vi "Open.vi"(4 "Gyro Full Scale Range":T8, 6 "Accel Full Scale Range":T9, 7 "I2C Channel":u8, 8 "error in (no error)":errorcluster, 9 "Clock Source":u8=1, 10 "Device Address":T10=104 items=["0x68"=104, "0x69"=105], 11 "LINX Resource":T1) -> (0 "error out":errorcluster, 3 "LINX Resource":T1)   [LabVIEW 2011, in "LINX-MPU60X0.lvlib"]
doc: "Initializes the MPU-60X0 device setting the clock source and the full ranges for the accelerometer and gyro."
uses:
  LINX-MPU60X0.lvlib
  AccelFullScaleRanges.ctl
  GyroFullScaleRanges.ctl
  <vilib>/LabVIEW Hacker/LINX/Private/Type Defs/Platform.ctl
  <vilib>/LabVIEW Hacker/LINX/Private/Type Defs/Interface.ctl
  <vilib>/LabVIEW Hacker/LINX/Private/Device/Type Defs/TCP Config.ctl
  <vilib>/LabVIEW Hacker/LINX/Private/Type Defs/Device Family.ctl
  <vilib>/LabVIEW Hacker/LINX/Private/Device/Type Defs/Channels.ctl
  <vilib>/LabVIEW Hacker/LINX/Private/Device/Type Defs/LINX Device Config.ctl
  <vilib>/LabVIEW Hacker/LINX/Private/Type Defs/LINX Ref.ctl
  DeviceAddresses.ctl
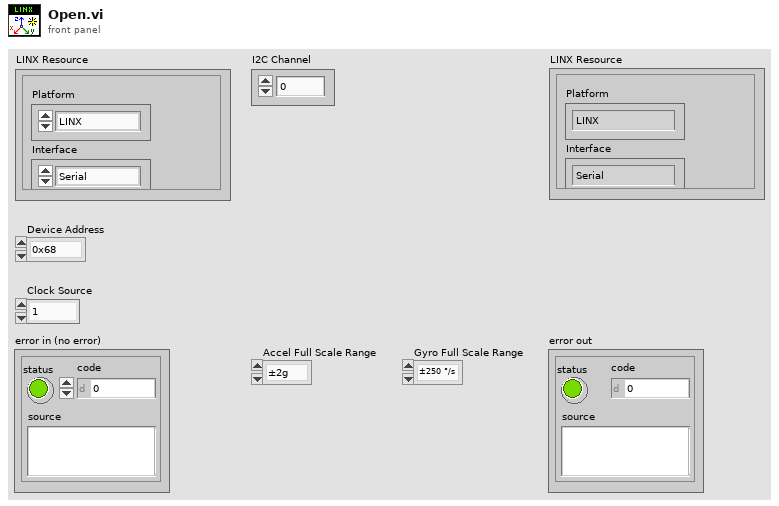
[diagram p1: front panel]
types:
  T1 = typedef "LVH-LINX.lvlib/LINX Ref.ctl" = cluster{"Platform":T2, "Interface":T3, "LINX Device Config":T4}
  T2 = typedef "LVH-LINX.lvlib/Platform.ctl" = enum16{"LINX", "myRIO"}
  T3 = typedef "LVH-LINX.lvlib/Interface.ctl" = enum16{"Serial", "TCP"}
  T4 = typedef "LVH-LINX.lvlib/Device.lvlib/LINX Device Config.ctl" = cluster{"Interface":T3, "COM Port":refnum<visa-resource-name>, "TCP Configuration":T5, "Device Family":T6, "Device ID":u8, "Device Name":string, "TCP Ref":refnum<k5>, "Channels":T7}
  T5 = typedef "LVH-LINX.lvlib/Device.lvlib/TCP Config.ctl" = cluster{"IP Address":string, "Port":u16}
  T6 = typedef "LVH-LINX.lvlib/Device Family.ctl" = enum8{"National Instruments", "Digilent", "Arduino"}
  T7 = typedef "LVH-LINX.lvlib/Channels.ctl" = cluster{"DI Channels":u8[], "DO Channels":u8[], "AI":u8[], "AO":u8[], "PWM":u8[], "QE":u8[], "UART":u8[], "I2C 2":u8[], "SPI":u8[], "CAN":u8[], "AI Ref (V)":dbl, "AO Resolution (Bits)":u8, "AO Ref (V)":dbl}
  T8 = typedef "LINX-MPU60X0.lvlib/GyroFullScaleRanges.ctl" = enum8{"±250 °/s", "±500 °/s", "±1000 °/s", "±2000 °/s"}
  T9 = typedef "LINX-MPU60X0.lvlib/AccelFullScaleRanges.ctl" = enum16{"±2g", "±4g", "±8g", "±16g"}
  T10 = typedef "LINX-MPU60X0.lvlib/DeviceAddresses.ctl" = u8
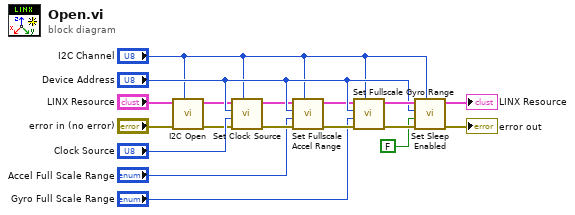
[diagram p0: block diagram]
diagram:
  n1 = call <vilib>:"I2C Open.vi"("I2C Channel (0)"="I2C Channel", "Error In"="error in (no error)", "LINX Resource"="LINX Resource") -> ("Error Out"=w2:errorcluster, "LINX Resource"=w4:T1)  [unwired: 7 in]
  n2 = call "Set Clock Source.vi"("I2C Channel"="I2C Channel", "error in (no error)"=w2, "Clock Source"="Clock Source", "Device Address"="Device Address", "LINX Resource"=w4) -> ("error out"=w16:errorcluster, "LINX Resource"=w8:T1)  [unwired: 5 in]
  n3 = call "Set Fullscale Accel Range.vi"("I2C Channel"="I2C Channel", "error in (no error)"=w16, "Accel Full Scale Range"="Accel Full Scale Range", "Device Address"="Device Address", "LINX Resource"=w8) -> ("error out"=w15:errorcluster, "LINX Resource"=w7:T1)  [unwired: 5 in]
  n4 = call "Set Fullscale Gyro Range.vi"("I2C Channel"="I2C Channel", "error in (no error)"=w15, "Gyro Full Scale Range"="Gyro Full Scale Range", "Device Address"="Device Address", "LINX Resource"=w7) -> ("error out"=w14:errorcluster, "LINX Resource"=w18:T1)  [unwired: 5 in]
  n5 = call "Set Sleep Enabled.vi"("I2C Channel"="I2C Channel", "error in (no error)"=w14, "Sleep?"=FALSE, "Device Address"="Device Address", "LINX Resource"=w18) -> ("error out"=→"error out":errorcluster, "LINX Resource"=→"LINX Resource":T1)  [unwired: 5 in]
